vi "release.vi"(8 "error in (no error)":errorcluster, 11 "InferEngineStruct":u64) -> (0 "error out":errorcluster)   [LabVIEW 2023]
uses:
  openvino_vi_wrapper.dll
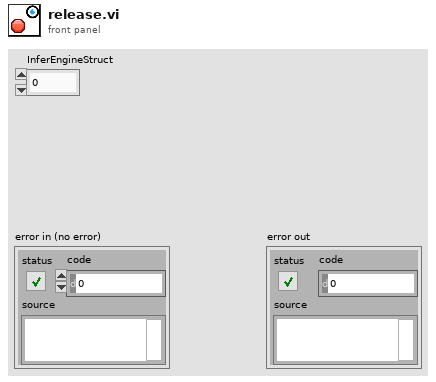
[diagram p1: front panel]
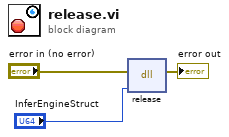
[diagram p0: block diagram]
diagram:
  n1 = dll-call lib="C:/Users/NUC/Desktop/LabVIEW_OpenVINO_Dll/yolov8_openvino_opensource/openvino_vi_wrapper/openvino_vi_wrapper.dll" fn="release"(error in="error in (no error)", "InferEngineStruct"="InferEngineStruct") -> (error out=→"error out":errorcluster)  [unwired: 4 in, 1 out]
